vi "v to p.vi"(11 "stop":bool) -> (0 "Output Variable":dbl format="%#_3e", 3 "output variable 2":dbl format="%#_3e")   [LabVIEW 2016]
uses:
  <vilib>/Analysis/baseanly.llb/Mean (DBL).vi
  <vilib>/Analysis/NI_AALBase.lvlib
panel:
  out "voltage 2":dbl format="%0.2f"
  out "voltage 1":dbl format="%0.2f"
  out "Array":dbl[][](array[numeric])
  out "data":dynamicdata(graph)
  out "Waveform Chart 2":dbl(graph)
  out "Waveform Chart":dbl(graph)
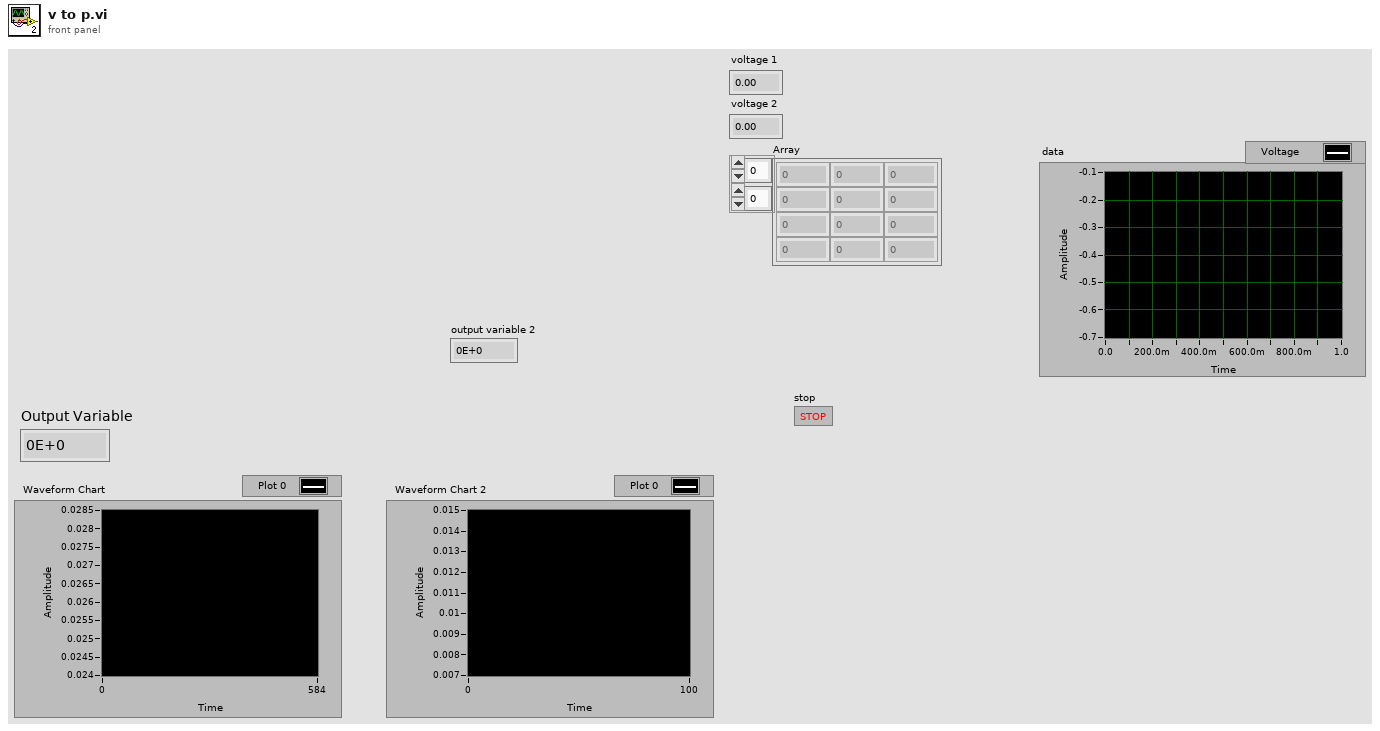
[diagram p1: front panel]
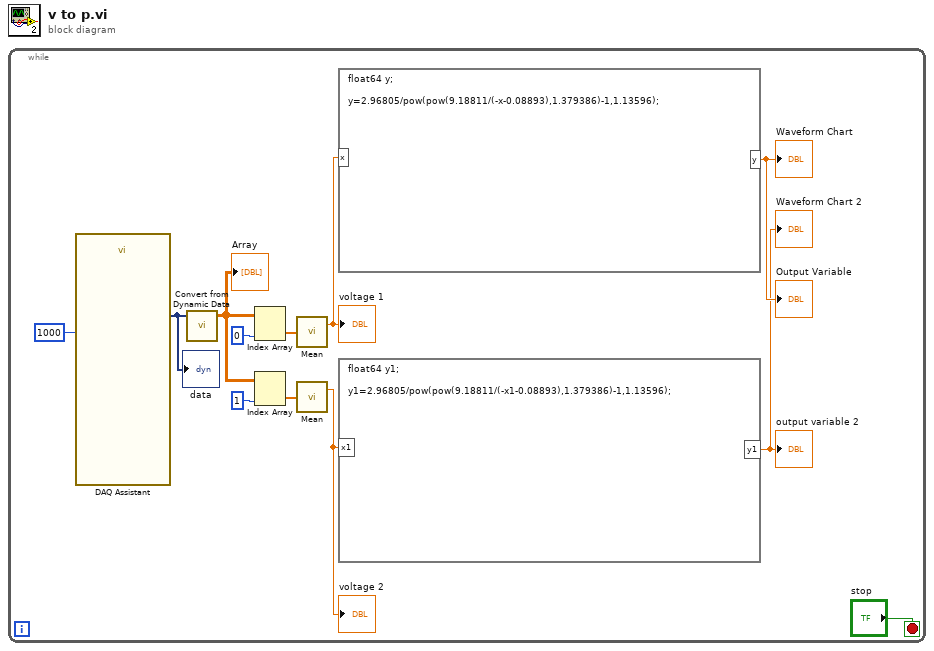
[diagram p0: block diagram]
diagram:
  n1 = while {
    stop <- "stop" stop-if-true
    n2 = call "DAQ Assistant"("number of samples"=1000) -> ("data"=w10:dynamicdata)  [unwired: 15 in, 3 out]
    "data" <- w10
    n3 = call "Convert from Dynamic Data"("Dynamic Data Type"=w10) -> ("Array"=w5:dbl[][])  [unwired: 3 in]
    "Array" <- w5
    n4 = Index Array(array=w5, index (col)=0 ("disabled index (col)")) -> (element=w7:dbl[])  [unwired: 1 in]
    n5 = Index Array(array=w5, index (col)=1 ("disabled index (col)")) -> (element=w4:dbl[])  [unwired: 1 in]
    n6 = call-poly <vilib>:"Mean.vi"("X"=w7) -> ("mean"=w3:dbl)  [unwired: 1 out]
    "voltage 1" <- w3
    n7 = call-poly <vilib>:"Mean.vi"("X"=w4) -> ("mean"=w2:dbl)  [unwired: 1 out]
    "voltage 2" <- w2
    n8 = formula code="float64 y;\n\ny=2.96805/pow(pow(9.18811/(-x-0.08893),1.379386)-1,1.13596);"("x"=w3) -> ("y"=→"Waveform Chart" →"Output Variable":dbl)
    n9 = formula code="float64 y1;\n\ny1=2.96805/pow(pow(9.18811/(-x1-0.08893),1.379386)-1,1.13596);"("x1"=w2) -> ("y1"=→"Waveform Chart 2" →"output variable 2":dbl)
  }
